vi "ConfigInterfaces.vi"(0 "reference in":refnum<class "Proccess.lvclass">, 5 "error in (no error)":errorcluster, 6 "Name":string, 7 "ConfigInterface":refnum<class "ConfigInterface.lvclass">, 8 "ParentName":string, 9 "MessageInterface":refnum<class "MessageInterface.lvclass">, 10 "Description":string, 11 "Logger":refnum<class "Logger.lvclass">) -> (14 "reference out":refnum<class "Proccess.lvclass">, 19 "error out":errorcluster)   [LabVIEW 2019, in "Proccess.lvclass"]
doc: "Constructor."
uses:
  Proccess.lvclass
  ConfigInterface_class/ConfigInterface.lvclass
  MessageInterface_class/MessageInterface.lvclass
  Logger_class/Logger.lvclass
  Proccess.lvclass/Proccess.ctl
  Logger_class/ObjData.ctl
  Logger_class/ObjType.ctl
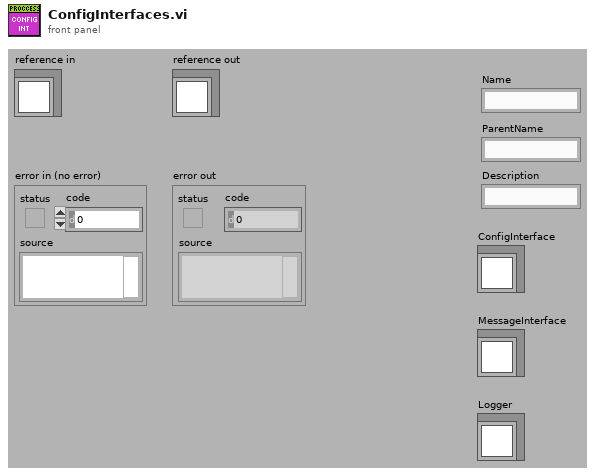
[diagram p1: front panel]
types:
  T1 = typedef "Logger.lvclass/ObjData.ctl" = cluster{"object_tag":string, "parent_tag":string, "object_type":T2, "description":string}
  T2 = typedef "Logger.lvclass/ObjType.ctl" = enum16{"Procces", "Device", "SignalA", "SignalD", "DI", "DO", "DA", "AI", "AO", "AA", "GUI"}
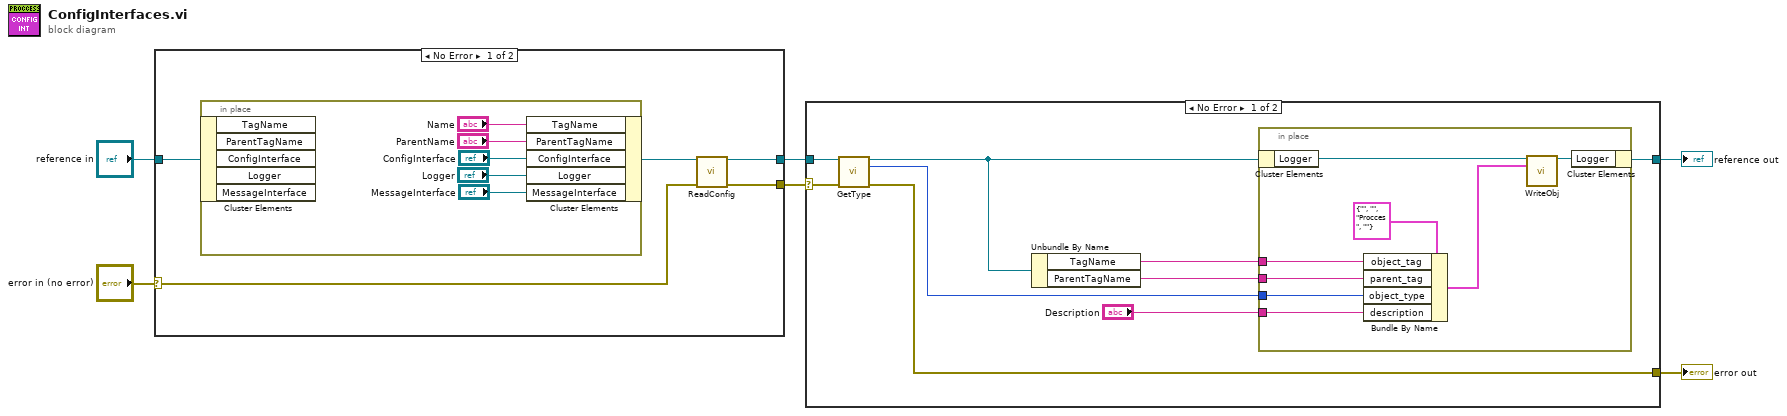
[diagram p0: block diagram]
diagram:
  n1 = case shown="No Error" "error in (no error)" {
    selector: "error in (no error)" -> [w10 w18]
    tunnel: [w8 w18] -> w3
    tunnel: [w9 w17] -> w4
    tunnel: "reference in" -> [w11 w17]
    frame No Error {
      n2 = in-place {
        n3 = in-place-cluster #1(w11) -> ()  [unwired: 5 out]
        n4 = in-place-cluster #1("TagName"="Name", "ParentTagName"="ParentName", "ConfigInterface"="ConfigInterface", "Logger"="Logger", "MessageInterface"="MessageInterface") -> (w7:refnum<class "Proccess.lvclass">)
      }
      n5 = call-dynamic "ReadConfig.vi"("reference in"=w7, "error in (no error)"=w10) -> ("reference out"=w9:refnum<class "Proccess.lvclass">, "error out"=w8:errorcluster)  [unwired: 12 in]
    }
    frame Error {
    }
  }
  n6 = case shown="No Error" w3 {
    selector: w3 -> [w23 w37]
    tunnel: [w27 w37] -> w1
    tunnel: [w20 w36] -> w2
    tunnel: w4 -> [w24 w36]
    frame No Error {
      n7 = call-dynamic "GetType.vi"("reference in"=w24, "error in (no error)"=w23) -> ("reference out"=w19:refnum<class "Proccess.lvclass">, "obj_type"=w22:T2, "error out"=w27:errorcluster)  [unwired: 11 in]
      n8 = Unbundle By Name(w19) -> ("TagName"=w26:string, "ParentTagName"=w25:string)
      n9 = in-place {
        in-place-border: w26 -> [w31]
        in-place-border: w25 -> [w30]
        in-place-border: w22 -> [w29]
        in-place-border: "Description" -> [w28]
        n10 = in-place-cluster #2(w19) -> ("Logger"=w34:refnum<class "Logger.lvclass">)
        n11 = Bundle By Name(cluster=T1 {"object_tag"="", "parent_tag"="", "object_type"=enum."Procces", "description"=""} ("device"), "object_tag"=w31, "parent_tag"=w30, "object_type"=w29, "description"=w28) -> (w32:T1)
        n12 = call "WriteObj.vi"("reference in"=w34, "device"=w32) -> ("reference out"=w33:refnum<class "Logger.lvclass">)  [unwired: 12 in, 1 out]
        n13 = in-place-cluster #2("Logger"=w33) -> (w20:refnum<class "Proccess.lvclass">)
      }
    }
    frame Error {
    }
  }
  "error out" <- w1
  "reference out" <- w2
